vi "Set Display Colours.vi"(8 "error in (no error)":errorcluster, 10 "Display Colours":T1, 11 "Main Display in":refnum<class "Main Display.lvclass">) -> (0 "error out":errorcluster, 3 "Main Display out":refnum<class "Main Display.lvclass">)   [LabVIEW 2016, in "Assert API Components.lvlib" / "Assert Display.lvlib" / "Main Display.lvlib" / "Main Display.lvclass"]
uses:
  Main Display.lvclass
  Display Colours.ctl
  Main Display.lvclass/Main Display.ctl
  Display Configurations/Base Display Configuration.lvclass/Base Display Configuration.ctl
  Display Configurations/Base Display Configuration.lvclass
  Main Display.lvlib
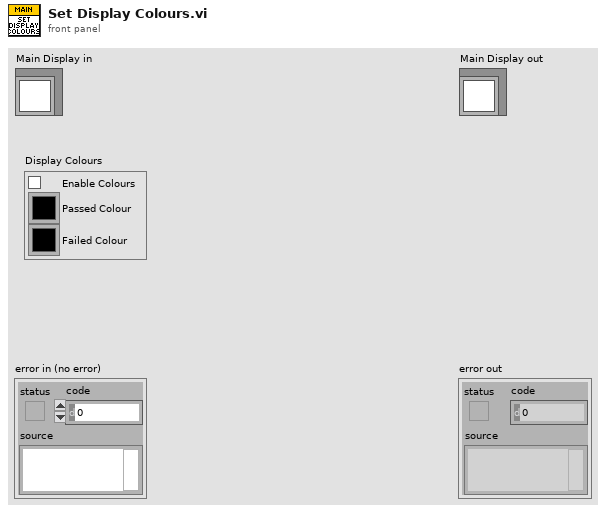
[diagram p1: front panel]
types:
  T1 = typedef "Assert API Components.lvlib/Assert Display.lvlib/Main Display.lvlib/Display Colours.ctl" = cluster{"Enable Colours":bool, "Passed Colour":u32, "Failed Colour":u32}
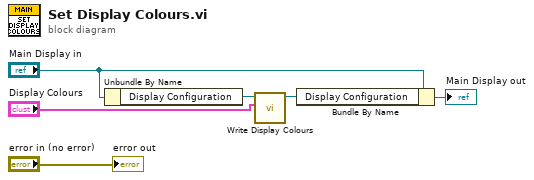
[diagram p0: block diagram]
diagram:
  n1 = Unbundle By Name("Main Display in") -> ("Display Configuration"=w4:refnum<class "Base Display Configuration.lvclass">)
  n2 = call "Write Display Colours.vi"("Display Colours"="Display Colours", "Base Display Configuration in"=w4) -> ("Base Display Configuration out"=w1:refnum<class "Base Display Configuration.lvclass">)  [unwired: 9 in]
  n3 = Bundle By Name(cluster="Main Display in", "Display Configuration"=w1) -> (→"Main Display out":refnum<class "Main Display.lvclass">)
  "error out" <- "error in (no error)"
